vi "Periodic Tasks.vi"(8 "error in":errorcluster) -> ()   [LabVIEW 2016]
doc: "This VI runs in parallel to other tasks. It can contain as many user-defined periodic loops as you need. These can carry out PID or other sorts of timed response."
uses:
  <vilib>/Rock Robotics/WPI/DriverStation/WPI_DriverStationRobotMode2.ctl
  <vilib>/Rock Robotics/WPI/Utilities/WPI_GetSetVariantRefNum.vi
  <vilib>/Rock Robotics/Network Tables/NT Write Number.vi
  <vilib>/Instr/_visa.llb/VISA Configure Serial Port (Instr).vi
  Systems/Global 1.vi
  Global 2.vi
panel:
  in  "reset gyro":bool
  out "Angle":dbl
  out "Waveform Chart":dbl(graph)
  out "PSI":dbl=101.0986199
  out "Right":dbl format="%#_13g"
  out "Left":dbl format="%#_13g"
  out "read buffer":string="B:2,X:203.00"
  in  "Search_Params":string[](array[string])=["B", "X", "Y", "W1", "H1", "W2", "H2"]
  out "Last Complete Message":string="B:2,X:203.00,Y:125.00,W1:11,H1:27,W2:8,H2:25"
  out "length":i32=44
  in  "off set":dbl format="%#_13g"
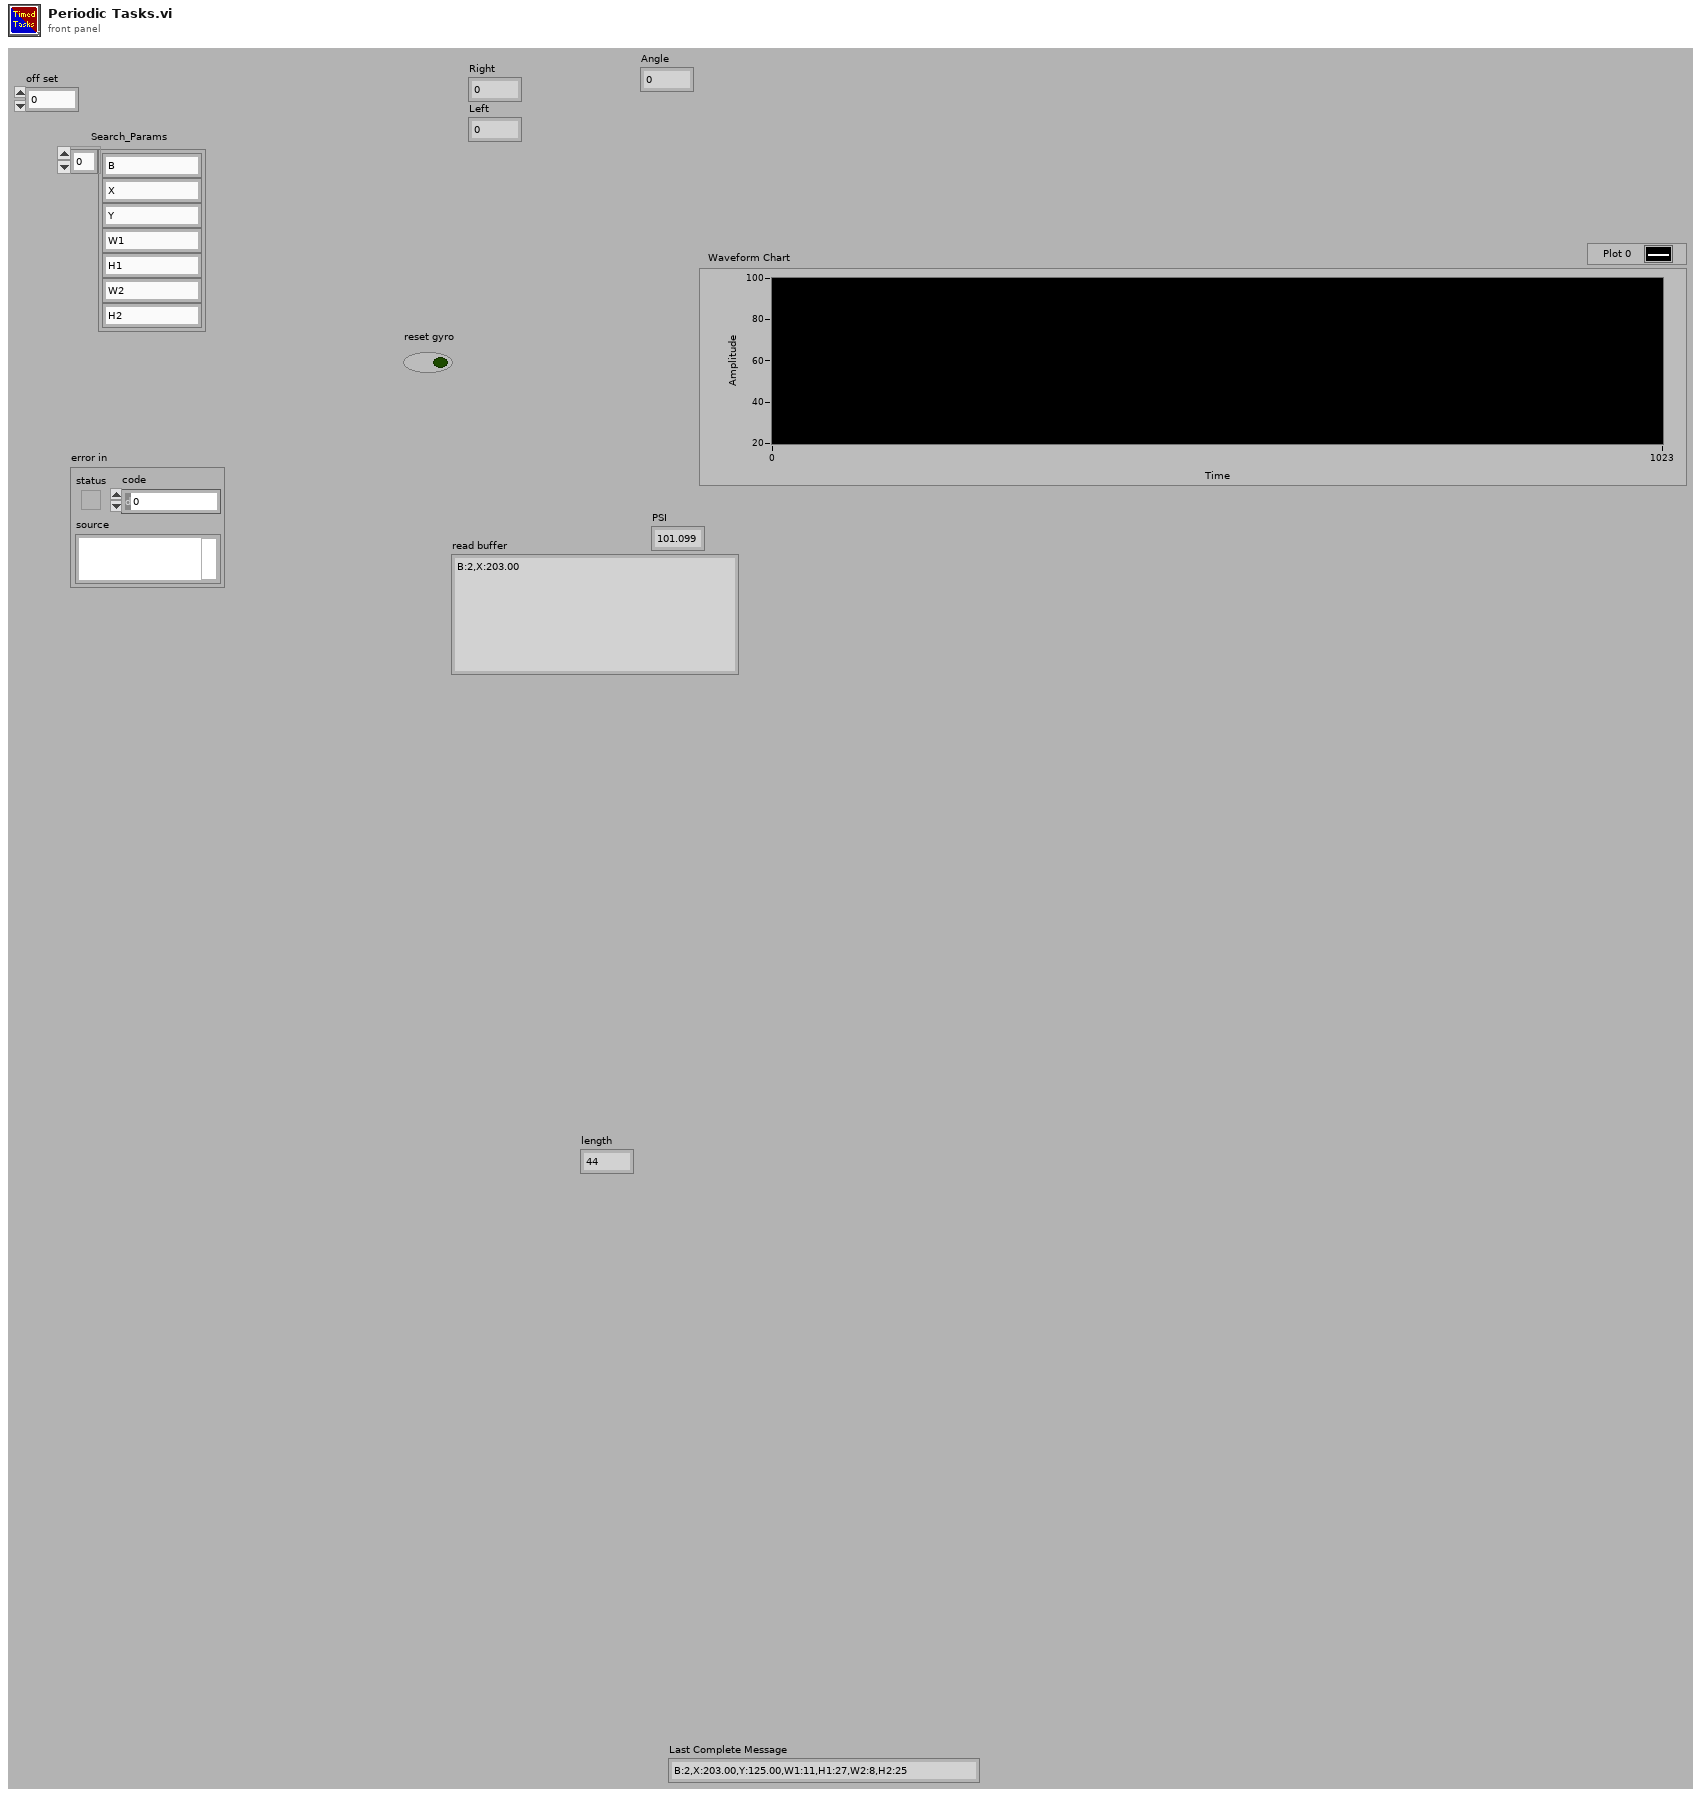
[diagram p1: front panel]
types:
  T1 = typedef "WPI_JoystickDevRef.ctl" = cluster{"Device":T2}
  T2 = typedef "WPI_JoystickDeviceEnum.ctl" = enum16{"USB 0", "USB 1", "USB 2", "USB 3", "USB 4", "USB 5"}
  T3 = typedef "WPI_AnalogChannelDevRef.ctl" = cluster{"DevStatus":errorcluster, "Analog Channel":T4}
  T4 = typedef "FPGA_AIChannel.ctl" = enum8{"AI 0", "AI 1", "AI 2", "AI 3", "AI MXP 0", "AI MXP 1", "AI MXP 2", "AI MXP 3", "Invalid"}
  T5 = typedef "WPI_MotorControlDeviceRef.ctl" = cluster{"DeviceStatus":errorcluster, "Type":T6, "PWM":cluster{"PWM Channel":T7, "DeadBand":T8}, "CAN":cluster{"Device Number":u8, "SetOutput VI Ref":variant, "GetOutput VI Ref":variant, "Enable VI Ref":variant, "Disable VI Ref":variant, "Data":variant}, "Invert":bool}
  T6 = typedef "WPI_MotorControlType.ctl" = enum16{"PWM", "CAN"}
  T7 = typedef "FPGA_DIOPWMChannel.ctl" = enum8{"PWM 0", "PWM 1", "PWM 2", "PWM 3", "PWM 4", "PWM 5", "PWM 6", "PWM 7", "PWM 8", "PWM 9", "PWM MXP 0", "PWM MXP 1", "PWM MXP 2", "PWM MXP 3", "PWM MXP 4", "PWM MXP 5", "PWM MXP 6", "PWM MXP 7", "PWM MXP 8", "PWM MXP 9", "Invalid"}
  T8 = typedef "WPI_PWMDeadband.ctl" = cluster{"Name":string, "maxPositivePwm":i32, "minPositivePwm":i32, "centerPwm":i32, "maxNegativePwm":i32, "minNegativePwm":i32, "angularRange":u16}
  T9 = typedef "WPI_GyroDevRef.ctl" = cluster{"DevStatus":errorcluster, "Analog Channel":T4, "Offset":dbl, "Gain (VoltsPerDegree/Second)":dbl, "Gyro Type":enum16{"Analog", "XRS450"}, "Handle":i32, "SPI Bus":T10, "Device Found":bool, "Sample Rate":dbl, "Calibrate On Open":bool}
  T10 = typedef "spi_bus.ctl" = enum16{"SPI On-Board, CS0", "SPI On-Board, CS1", "SPI On-Board, CS2", "SPI On-Board, CS3", "SPI MXP", "Invalid"}
  T11 = typedef "WPI_DriverStationRobotMode2.ctl" = enum16{"Autonomous Disabled", "Autonomous Enabled", "Teleop Disabled", "Teleop Enabled", "Disconnected", "Finish", "Test Disabled", "Test Enabled", "Emergency Stopped"}
  T12 = typedef "WPI_CANTalonSRX_GlobalStatus.ctl" = cluster{"Applied Throttle":dbl, "Module Enabled":bool, "CAN Error":errorcluster, "Closed Loop Error":dbl, "Forward Limit Switch Closed":bool, "Reverse Limit Switch Closed":bool, "Sensor Position":dbl, "Sensor Velocity":dbl, "Current":dbl, "Sticky Fault - Over Temp":bool, "Sticky Fault - Under Voltage":bool, "Sticky Fault - Forward Limit":bool, "Sticky Fault - Reverse Limit":bool, "Sticky Fault - Forward Soft Limit":bool, "Sticky Fault - Reverse Soft Limit":bool, "Brake is Enabled":bool, "Encoder Position":dbl, "Encoder Velocity":dbl, "Encoder Index Count":dbl, "Encoder A Pin State":bool, "Encoder B Pin State":bool, "Encoder Index Pin State":bool, "Analog In":dbl, "Analog In Velocity":dbl, "Temperature (C)":dbl, "Battery Voltage":dbl, "Control 5 Is Supported":bool, "Current Profile Slot Select":dbl, "Pos Div 8":bool, "Vel Div 4":bool, "Pulse Width Position":i32, "Pulse Width Velocity":i32, "Pulse Width Rise To Rise (us)":i32, "Pulse Width Rise To Fall (us)":i32, "Mot Prof Active Is Under Run":bool, "Mot Prof Active Has Under Run":bool, "Mot Prof Active Is Last":bool, "Mot Prof Active Velocity Only":bool, "Mot Prof Active Is Valid":bool, "Mot Prof Buffer Is Full":bool, "Mot Prof Active Profile Slot Select":i32, "Mot Prof NextID":i32, "Mot Prof Count":i32, "Mot Prof Active Velocity":dbl, "Mot Prof Active Position":dbl, "Mot Prof Output Enable":i32}
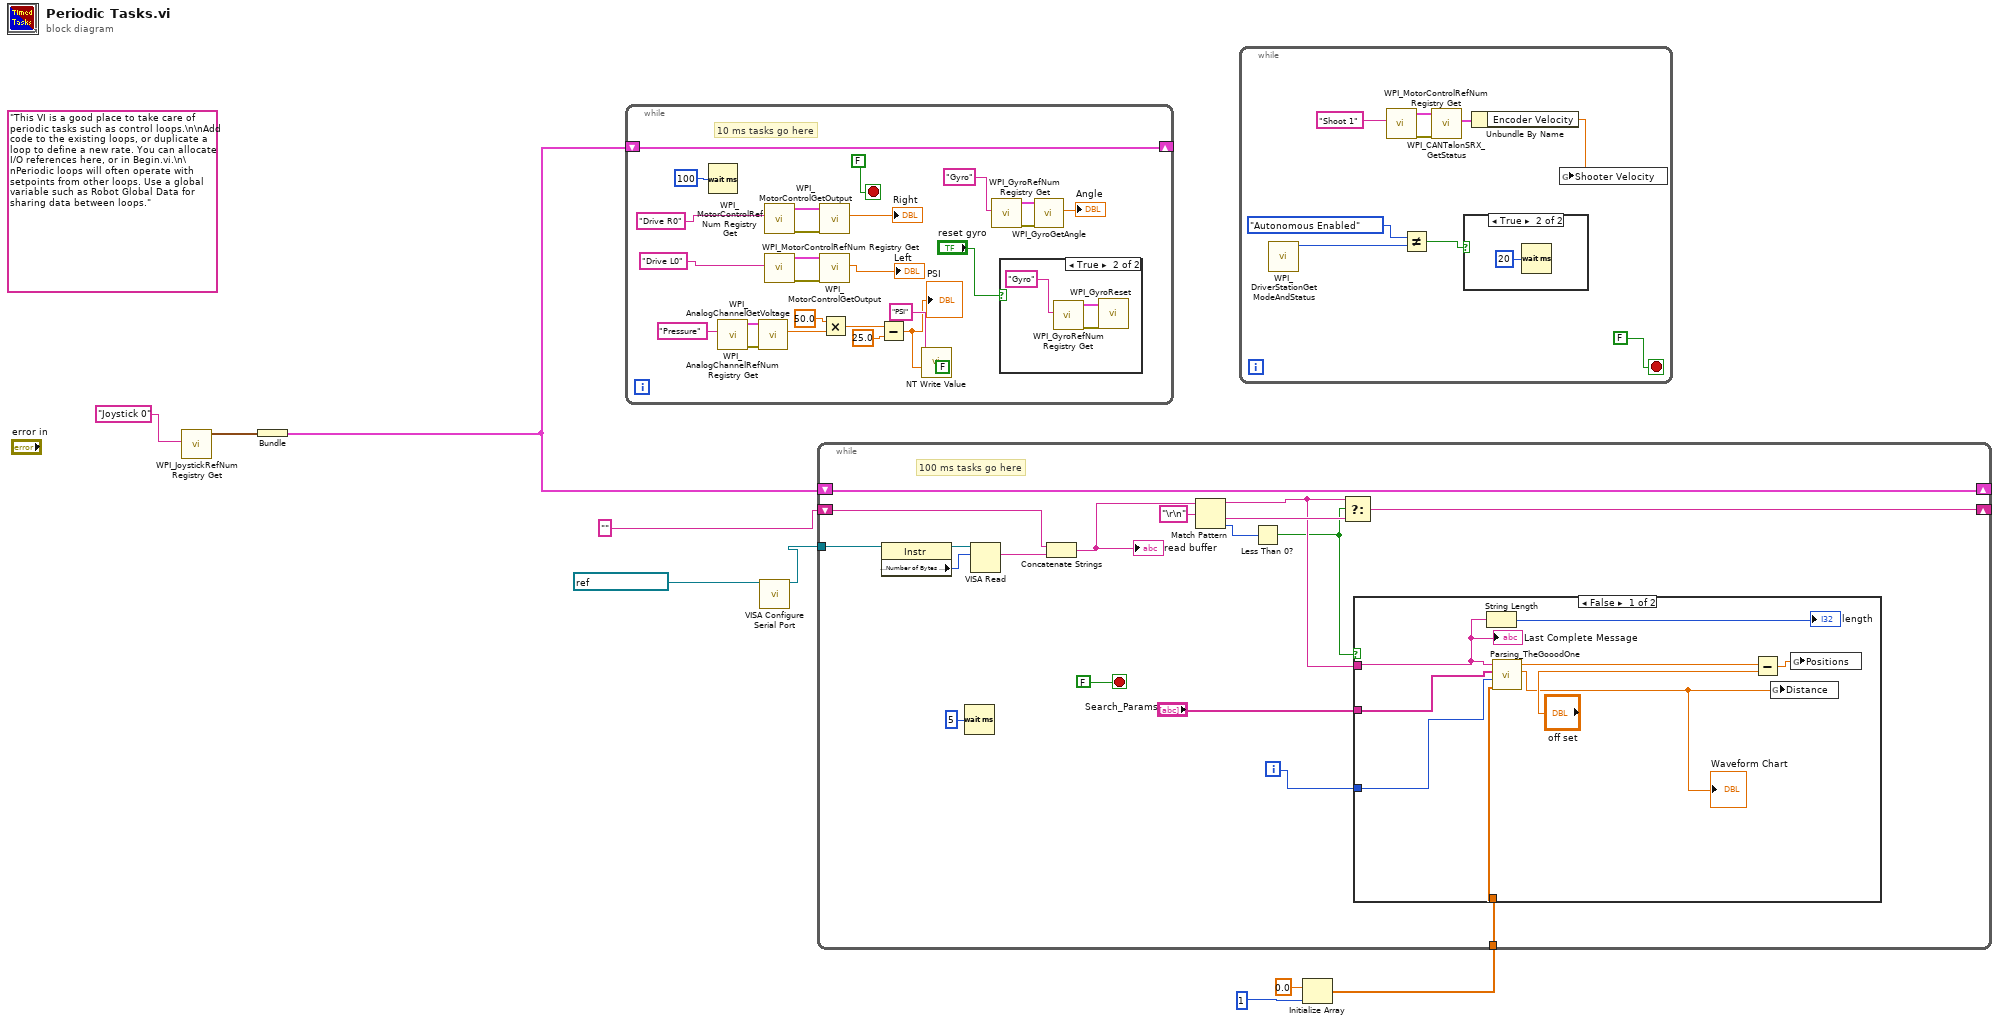
[diagram p0: block diagram]
diagram:
  (unwired) "This VI is a good place to take care of periodic tasks such as control loops.\n\nAdd code to the existing loops, or duplicate a loop to define a new rate. You can allocate I/O references here, or in Begin.vi.\n\nPeriodic loops will often operate with setpoints from other loops. Use a global variable such as Robot Global Data for sharing data between loops."
  n1 = call <vilib>:"WPI_JoystickRefNum Registry Get.vi"("refnum name"="Joystick 0") -> ("JoystickDevRef"=w2:T1)  [unwired: 1 in, 9 out]
  n2 = Bundle("JoystickDevRef"=w2) -> (w3:cluster{"JoystickDevRef":T1})  [unwired: 1 out]
  n3 = while {
    shift-right: [w32] -> _
    shift-left: w3 -> [w32]
    stop <- FALSE stop-if-true
    (unwired) FALSE
    # "10 ms tasks go here"
    n4 = Wait (ms)(milliseconds to wait=u32 100) -> ()  [unwired: 1 out]
    n5 = call <vilib>:"WPI_AnalogChannelRefNum Registry Get.vi"("refnum name"="Pressure") -> ("error out"=w25:errorcluster, "AIDeviceRef"=w24:T3)  [unwired: 9 in]
    n6 = call <vilib>:"WPI_AnalogChannelGetVoltage.vi"("error in (no error)"=w25, "AIDeviceRef"=w24) -> ("Voltage"=w22:dbl)  [unwired: 7 in, 2 out]
    n7 = call <vilib>:"WPI_MotorControlRefNum Registry Get.vi"("refnum name"="Drive R0") -> ("error out"=w29:errorcluster, "MotorControlDevRef"=w31:T5)  [unwired: 9 in]
    n8 = call <vilib>:"WPI_MotorControlRefNum Registry Get.vi"("refnum name"="Drive L0") -> ("error out"=w28:errorcluster, "MotorControlDevRef"=w30:T5)  [unwired: 9 in]
    n9 = call <vilib>:"WPI_MotorControlGetOutput.vi"("error in"=w29, "MotorControlDevRef"=w31) -> ("Output"=→"Right":dbl)  [unwired: 7 in, 2 out]
    n10 = call <vilib>:"WPI_MotorControlGetOutput.vi"("error in"=w28, "MotorControlDevRef"=w30) -> ("Output"=→"Left":dbl)  [unwired: 7 in, 2 out]
    n11 = Multiply(x=50.0, y=w22) -> (x*y=w20:dbl)
    n12 = Subtract(x=w20, y=25.0) -> (x-y=w17:dbl)
    "PSI" <- w17
    n13 = call-poly <vilib>:"NT Write Value.vi"("Numeric"=w17, "Name"="PSI") -> ()  [unwired: 9 in, 1 out]
    n14 = call <vilib>:"WPI_GyroRefNum Registry Get.vi"("refnum name"="Gyro") -> ("error out"=w14:errorcluster, "GyroDevRef"=w13:T9)  [unwired: 9 in]
    n15 = case shown="True" "reset gyro" {
      frame False {
      }
      frame True {
        n16 = call <vilib>:"WPI_GyroRefNum Registry Get.vi"("refnum name"="Gyro") -> ("error out"=w36:errorcluster, "GyroDevRef"=w35:T9)  [unwired: 9 in]
        n17 = call <vilib>:"WPI_GyroReset.vi"("error in"=w36, "GyroDevRef"=w35) -> ()  [unwired: 8 in, 2 out]
      }
    }
    n18 = call <vilib>:"WPI_GyroGetAngle.vi"("error in"=w14, "GyroDevRef"=w13) -> ("Angle"=→"Angle":dbl)  [unwired: 5 in, 4 out]
  }
  n19 = call-poly "VISA Configure Serial Port"("VISA resource name"=refnum<visa-resource-name> "ASRL2::INSTR") -> ("VISA resource name out"=w5:refnum<visa-resource-name>)  [unwired: 13 in, 1 out]
  n20 = while {
    stop <- FALSE stop-if-true
    n21 = call <vilib>:"WPI_DriverStationGetModeAndStatus.vi"() -> ("Robot Mode"=w40:T11)  [unwired: 10 in, 1 out]
    n22 = call <vilib>:"WPI_MotorControlRefNum Registry Get.vi"("refnum name"="Shoot 1") -> ("error out"=w44:errorcluster, "MotorControlDevRef"=w45:T5)  [unwired: 9 in]
    n23 = Not Equal?(x=WPI_DriverStationRobotMode2."Autonomous Enabled" ("Robot Mode"), y=w40) -> (x != y?=w38:bool)
    n24 = call <vilib>:"WPI_CANTalonSRX_GetStatus.vi"("error in (no error)"=w44, "CAN Talon SRX Ref"=w45) -> ("Talon SRX Status"=w43:T12)  [unwired: 7 in, 2 out]
    n25 = case shown="True" w38 {
      frame False {
      }
      frame True {
        n26 = Wait (ms)(milliseconds to wait=u32 20) -> ()  [unwired: 1 out]
      }
    }
    n27 = Unbundle By Name(w43) -> ("Encoder Velocity"=w42:dbl)
    n28 = global write "Global 2.vi" "Shooter Velocity"(w42) -> ()
  }
  n29 = Initialize Array(0.0 ("element"), 1) -> (w9:dbl[])
  n30 = while {
    shift-right: [w64] -> _
    shift-left: w3 -> [w64]
    tunnel: w5 -> [w59]
    shift-right: [w51] -> _
    shift-left: "" -> [w58]
    tunnel: w9 -> [w48]
    i -> [w49]
    stop <- FALSE stop-if-true
    # "100 ms tasks go here"
    n31 = property class="Instr"(reference=w59) -> (reference out=w63:refnum<visa-resource-name>, "Serial Settings:Number of Bytes at Serial Port"=w62:u32)  [unwired: 1 in, 1 out]
    n32 = Wait (ms)(milliseconds to wait=u32 5) -> ()  [unwired: 1 out]
    n33 = VISA Read(VISA resource name=w63, byte count=w62) -> (read buffer=w57:string)  [unwired: 1 in, 3 out]
    n34 = Concatenate Strings(w58, w57) -> (w56:string)
    "read buffer" <- w56
    n35 = Match Pattern(string=w56, regular expression="\r\n") -> (before substring=w52:string, after substring=w53:string, offset past match=w54:i32)  [unwired: 1 in, 1 out]
    n36 = Less Than 0?(x=w54) -> (x < 0?=w50:bool)
    n37 = Select(t=w52, s=w50, f=w53) -> (s? t:f=w51:string)
    n38 = case shown="False" w50 {
      tunnel: "Search_Params" -> [w73 _]
      tunnel: w52 -> [w72 _]
      tunnel: w49 -> [w68 _]
      tunnel: w48 -> [w67 _]
      frame False {
        n39 = String Length(string=w72) -> (length=→"length":i32)
        n40 = call "Parsing_TheGooodOne.vi"("array"=w67, "Iterations"=w68, "Search_Params"=w73, "Input"=w72) -> ("Corrected distance"=w66:dbl, "Value-Reference"=w71:dbl)  [unwired: 4 in]
        "Waveform Chart" <- w66
        n41 = Subtract(x=w71, y="off set") -> (x-y=w69:dbl)
        n42 = global write "Global 1.vi" "Distance"(w66) -> ()
        n43 = global write "Global 1.vi" "Positions"(w69) -> ()
        "Last Complete Message" <- w72
      }
      frame True {
      }
    }
  }
